vi "Send Command.vi"(8 "error in (no error)":errorcluster, 9 "timeout in ms (0)":i32 format="%d ms", 10 "command":T1, 11 "Dispatcher in":refnum<class "Dispatcher Thread.lvclass">) -> (0 "error out":errorcluster, 1 "timed out?":bool, 3 "Dispatcher out":refnum<class "Dispatcher Thread.lvclass">)   [LabVIEW 2017, in "DSF Core.lvlib" / "Dispatcher Thread.lvclass"]
uses:
  Dispatcher Thread.lvclass
  Interfaces/Dispatcher/Command Data.ctl
  Interfaces/Dispatcher/Command.ctl
  Interfaces/Dispatcher/Parameters.ctl
  Dispatcher Thread.lvclass/Dispatcher Thread.ctl
  Interfaces/Interface/Interface.lvclass/Interface.ctl
  Debug/FIFO Flags/FIFO Flags.lvclass/FIFO Flags.ctl
  Interfaces/Dispatcher/Write Dispatcher Command.vi
  Interfaces/Interface/Write Command.vi
  Interfaces/Interface/Get Command FIFO.vi
  Interfaces/Interface/Write RT FIFO(16B).vi
  Interfaces/Interface/Get Debug Flags.vi
  Debug/FIFO Flags/Get Infinite Timeouts.vi
  Interfaces/Dispatcher/Dispatcher Interface.lvclass
  C:/Git/DSF/Data Sharing Framework/Source/Core/Engine/Classes/Interfaces/Interface/Interface.lvclass
  Interfaces/Interface/Errors.vi
  Interfaces/Interface/Command Timeout.vi
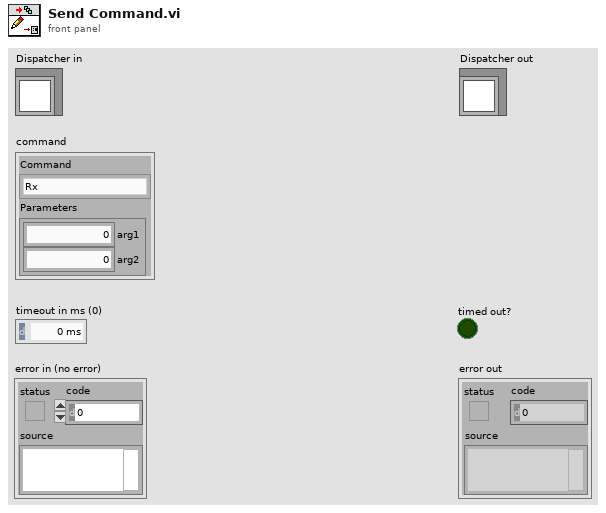
[diagram p1: front panel]
types:
  T1 = typedef "DSF Core.lvlib/Dispatcher Interface.lvclass/Command Data.ctl" = cluster{"Command":T2, "Parameters":T3}
  T2 = typedef "DSF Core.lvlib/Dispatcher Interface.lvclass/Command.ctl" = enum8{"Rx", "Tx", "Shutdown"}
  T3 = typedef "DSF Core.lvlib/Dispatcher Interface.lvclass/Parameters.ctl" = cluster{"arg1":u64, "arg2":u64}
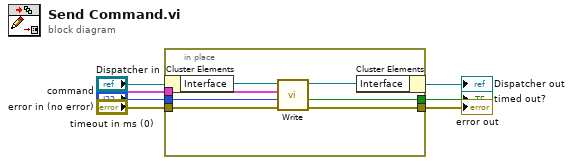
[diagram p0: block diagram]
diagram:
  n1 = in-place {
    in-place-border: "error in (no error)" -> [w12]
    in-place-border: [w11] -> w5
    in-place-border: "timeout in ms (0)" -> [w10]
    in-place-border: "command" -> [w9]
    in-place-border: [w8] -> w2
    n2 = in-place-cluster #1("Dispatcher in") -> ("Interface"=w14:refnum<class "Dispatcher Interface.lvclass">)
    n3 = call-poly "Write.vi"("error in (no error)"=w12, "timeout in ms (0)"=w10, "command"=w9, "Dispatcher Interface in"=w14) -> ("error out"=w11:errorcluster, "timed out?"=w8:bool, "Dispatcher Interface out"=w13:refnum<class "Dispatcher Interface.lvclass">)  [unwired: 5 in]
    n4 = in-place-cluster #1("Interface"=w13) -> (→"Dispatcher out":refnum<class "Dispatcher Thread.lvclass">)
  }
  "error out" <- w5
  "timed out?" <- w2
